vi "PH_PSDBWriter.get Subsystem DIM Service.vi"(1 "no link":bool, 2 "typeDescriptor":string, 3 "data":i8[](array[numeric]), 4 "quality":i32) -> (0 "PHELIX Subsystems":T1 items=["Miscellaneous", "fs-Frontend", "ns-Frontend", "PreAmp", "MainAmp", "MAS", "COS", "Beamline", "Experiment Laserbay", "Experiment Laserlabor", "Experiment Z6", "Timing", "Pulsed Power"])   [LabVIEW 2014, in "PH_PSDBWriter.lvlib"]
uses:
  PH_PSDBWriter.lvlib
  PH_PSDBWriter.PHELIX-Subsystems.ctl
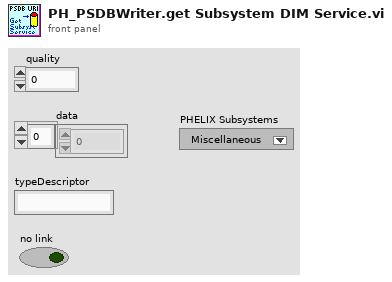
[diagram p1: front panel]
types:
  T1 = typedef "PH_PSDBWriter.lvlib/PH_PSDBWriter.PHELIX-Subsystems.ctl" = i32
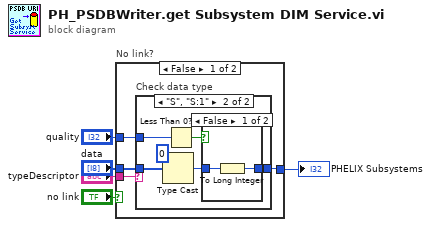
[diagram p0: block diagram]
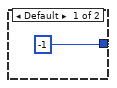
[diagram p2: hidden frame]
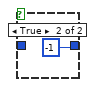
[diagram p3: hidden frame]
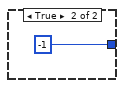
[diagram p4: hidden frame]
diagram:
  n1 = case "No link?" shown="False" "no link" {
    tunnel: [w9 -1] -> w5
    tunnel: "quality" -> [w8 _]
    tunnel: "data" -> [w7 _]
    tunnel: "typeDescriptor" -> [w6 _]
    frame False {
      n2 = case "Check data type" shown="\"S\", \"S:1\"" w6 {
        tunnel: [-1 w16] -> w9
        tunnel: w8 -> [_ w14]
        tunnel: w7 -> [_ w12]
        frame Default {
        }
        frame "S", "S:1" {
          n3 = Type Cast(type=i16 0, x=w12) -> (*(type *) &x=w11:i16)
          n4 = Less Than 0?(x=w14) -> (x < 0?=w15:bool)
          n5 = case shown="False" w15 {
            tunnel: [w17 -1] -> w16
            tunnel: w11 -> [w18 _]
            frame False {
              n6 = To Long Integer(number=w18) -> (32bit integer=w17:i32)
            }
            frame True {
            }
          }
        }
      }
    }
    frame True {
    }
  }
  "PHELIX Subsystems" <- w5
